vi "Sample_SimpleCoERead.vi"() -> ()   [LabVIEW 2022 SP3, in "EtherCAT_Library.lvlib"]
uses:
  EtherCAT_Library.lvlib
  <userlib>/Beckhoff-LabVIEW-Interface/_DependsOn/TypeDefs/Utilities/CoE Object Entry.ctl
  <userlib>/Beckhoff-LabVIEW-Interface/_DependsOn/TypeDefs/Utilities/CoE Object DataType.ctl
panel:
  out "output cluster":T3 {"Object Entry"."Index" format="%x"; "Object Entry"."SubIndex" format="%x"; "Object Entry"."DataType" items=["UNDEFINED"=0, "BOOLEAN"=1, "INTEGER8"=2, "INTEGER16"=3, "INTEGER32"=4, "UNSIGNED8"=5, "UNSIGNED16"=6, "UNSIGNED32"=7, "REAL32"=8, "VISIBLE_STRING"=9, "OCTET_STRING"=10, "UNICODE_STRING"=11, "TIME_OF_DAY"=12, "TIME_DIFFERENCE"=13, "DOMAIN"=15, "INTEGER24"=16, "REAL64"=17, "INTEGER40"=18, "INTEGER48"=19, "INTEGER56"=20, "INTEGER64"=21, "UNSIGNED40"=23, "UNSIGNED48"=24, "UNSIGNED56"=25, "UNSIGNED64"=26, "GUID"=29, "BYTE"=30, "BITARR8"=45, "BITARR16"=46, "BITARR32"=47, "PDO_MAPPING"=33, "IDENTITY"=35, "COMMAND_PAR"=37, "SYNC_PAR"=41, "BIT1"=48, "BIT2"=49, "BIT3"=50, "BIT4"=51, "BIT5"=52, "BIT6"=53, "BIT7"=54, "BIT8"=55, "ENUM"=2048]}
  in  "Device address":string="10.97.0.23.2.1:1007"
  in  "Index":u16=32768 format="%x"
  in  "SubIndex":u8=1 format="%x"
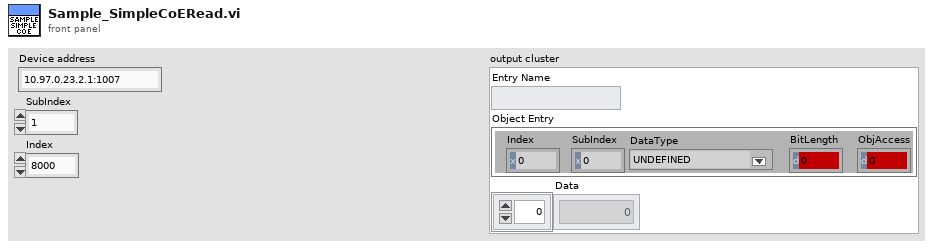
[diagram p1: front panel]
types:
  T1 = typedef "CoE Object Entry.ctl" = cluster{"Index":u16, "SubIndex":u8, "ValueInfo":u8, "DataType":T2, "BitLength":u16, "ObjAccess":u16}
  T2 = typedef "CoE Object DataType.ctl" = u16
  T3 = cluster{"Entry Name":string, "Object Entry":T1, "Data":u8[]}
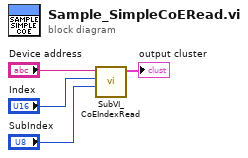
[diagram p0: block diagram]
diagram:
  n1 = call "SubVI_CoEIndexRead.vi"("SubIndex"="SubIndex", "Index"="Index", "Device address"="Device address") -> ("output cluster"=→"output cluster":T3)  [unwired: 7 in, 1 out]
